vi "Assign LS Slave Timing.vi"(8 "error in (no error)":errorcluster, 10 "MasterTimingInfo":T1, 11 "DAQ Task in":refnum<class "DAQ Task.lvclass">) -> (0 "error out":errorcluster, 3 "DAQ Task out":refnum<class "DAQ Task.lvclass">)   [LabVIEW 2012, in "Data Acquisition.lvlib" / "DAQ Task.lvclass"]
uses:
  DAQ Task.lvclass
  Controls/Master Timing Info.ctl
  DAQ Task.lvclass/DAQ Task.ctl
  <vilib>/DAQmx/configure/trigger.llb/DAQmx Start Trigger (Digital Edge).vi
  <resource>/objmgr/daqmx.rc
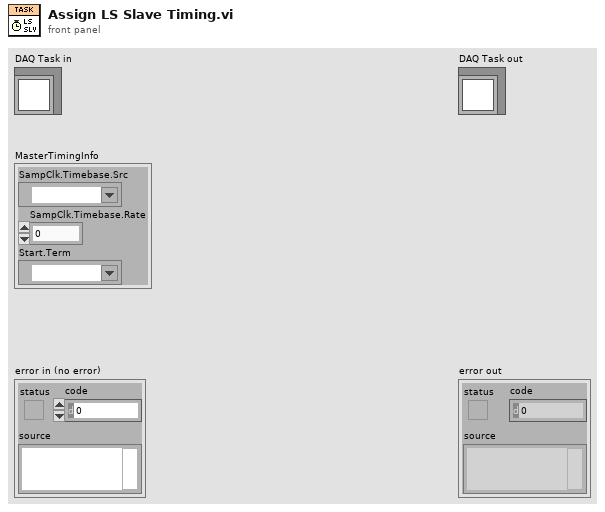
[diagram p1: front panel]
types:
  T1 = typedef "Data Acquisition.lvlib/DAQ Task.lvclass/Master Timing Info.ctl" = cluster{"SampClk.Timebase.Src":tag, "SampClk.Timebase.Rate":dbl, "Start.Term":tag}
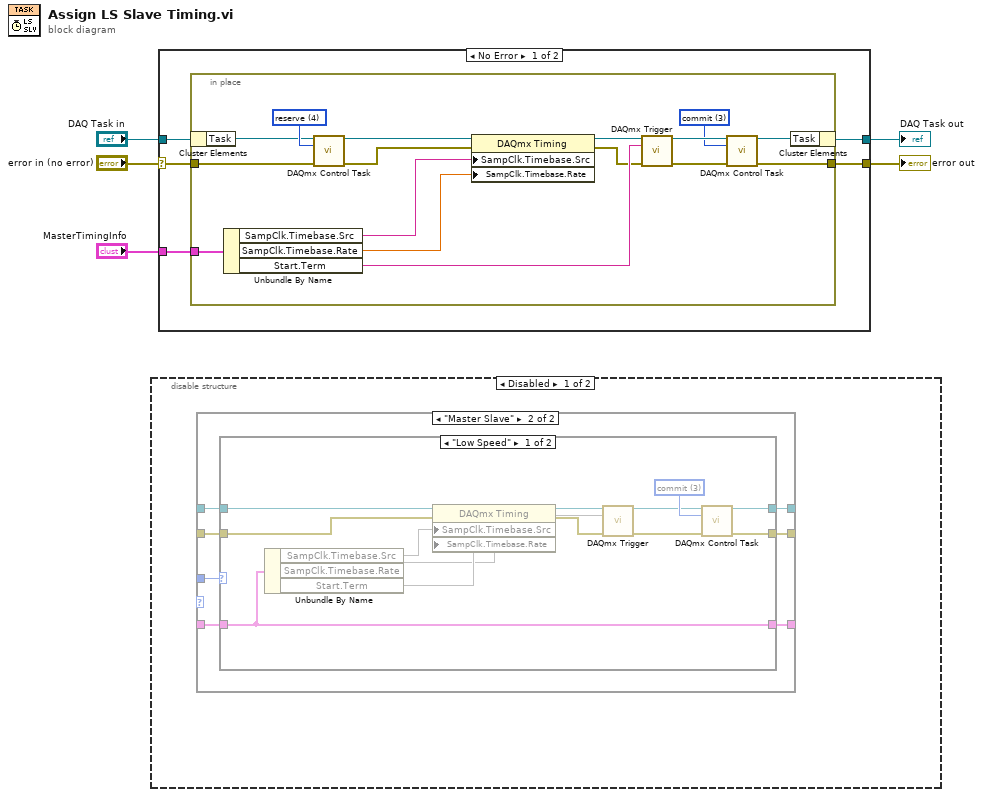
[diagram p0: block diagram]
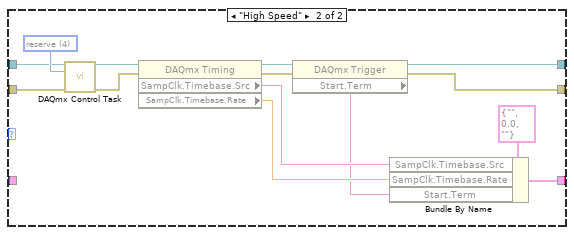
[diagram p3: hidden frame]
diagram:
  n1 = disable-structure shown="Disabled" {
    frame Disabled {
      n2 = case shown="\"Master Slave\"" {
        selector: _ -> [_ _]
        tunnel: [w7 w15] -> _
        tunnel: _ -> [w6 w14]
        tunnel: [w6 w13] -> _
        tunnel: _ -> [w8 w12]
        tunnel: _ -> [w7 w11]
        tunnel: [w8 w10] -> _
        tunnel: _ -> [_ w9]
        frame Default {
        }
        frame "Master Slave" {
          n3 = case shown="\"Low Speed\"" w9 {
            tunnel: w12 -> [w20 w41]
            tunnel: w11 -> [w19 w40]
            tunnel: [w18 w39] -> w10
            tunnel: [w17 w38] -> w15
            tunnel: [w16 w29] -> w13
            tunnel: w14 -> [w16 _]
            frame "Low Speed" {
              w28 = 3 items=["verify"=2, "reserve"=4, "commit"=3, "unreserve"=5, "abort"=6] ("action")
              n4 = Unbundle By Name(w16) -> ("SampClk.Timebase.Src"=w23, "SampClk.Timebase.Rate"=w21, "Start.Term"=w22)
              n5 = property class="DAQmx Timing"(reference=w20, error in=w19, "SampClk.Timebase.Src"=w23, "SampClk.Timebase.Rate"=w21) -> (reference out=w25:refnum<k21>, error out=w24:errorcluster)
              n6 = call-poly <vilib>:"DAQmx Trigger.vi"("task/channels in"=w25, "source"=w22, "error in"=w24) -> ("task out"=w27:refnum<k21>, "error out"=w26:errorcluster)  [unwired: 11 in]
              n7 = call <vilib>:"DAQmx Control Task.vi"("task/channels in"=w27, "action"=w28, "error in"=w26) -> ("task out"=w18:refnum<k21>, "error out"=w17:errorcluster)  [unwired: 11 in]
            }
            frame "High Speed" {
              w42 = 4 items=["verify"=2, "reserve"=4, "commit"=3, "unreserve"=5, "abort"=6] ("action")
              n8 = call <vilib>:"DAQmx Control Task.vi"("task/channels in"=w41, "action"=w42, "error in"=w40) -> ("task out"=w37:refnum<k21>, "error out"=w34:errorcluster)  [unwired: 11 in]
              n9 = property class="DAQmx Timing"(reference=w37, error in=w34) -> (reference out=w36:refnum<k21>, error out=w35:errorcluster, "SampClk.Timebase.Src"=w32:tag, "SampClk.Timebase.Rate"=w31:dbl)
              n10 = property class="DAQmx Trigger"(reference=w36, error in=w35) -> (reference out=w39:refnum<k21>, error out=w38:errorcluster, "Start.Term"=w30:tag)
              n11 = Bundle By Name(cluster=T1 {"SampClk.Timebase.Src"="", "SampClk.Timebase.Rate"=0.0, "Start.Term"=""} ("MasterTimingInfo"), "SampClk.Timebase.Src"=w32, "SampClk.Timebase.Rate"=w31, "Start.Term"=w30) -> (w29:T1)
            }
          }
        }
      }
    }
    frame Enabled {
    }
  }
  n12 = case shown="No Error" "error in (no error)" {
    selector: "error in (no error)" -> [w43 w65]
    tunnel: [w47 w65] -> w5
    tunnel: [w45 w64] -> w4
    tunnel: "DAQ Task in" -> [w44 w64]
    tunnel: "MasterTimingInfo" -> [w46 _]
    frame No Error {
      n13 = in-place {
        in-place-border: [w52] -> w47
        in-place-border: w46 -> [w51]
        in-place-border: w43 -> [w50]
        w55 = 3 items=["verify"=2, "reserve"=4, "commit"=3, "unreserve"=5, "abort"=6] ("action")
        w63 = 4 items=["verify"=2, "reserve"=4, "commit"=3, "unreserve"=5, "abort"=6] ("action")
        n14 = in-place-cluster #1(w44) -> ("Task"=w49:refnum<k21>)
        n15 = Unbundle By Name(w51) -> ("SampClk.Timebase.Src"=w60:tag, "SampClk.Timebase.Rate"=w62:dbl, "Start.Term"=w61:tag)
        n16 = call <vilib>:"DAQmx Control Task.vi"("task/channels in"=w49, "action"=w63, "error in"=w50) -> ("task out"=w54:refnum<k21>, "error out"=w53:errorcluster)  [unwired: 11 in]
        n17 = property class="DAQmx Timing"(reference=w54, error in=w53, "SampClk.Timebase.Src"=w60, "SampClk.Timebase.Rate"=w62) -> (reference out=w58:refnum<k21>, error out=w59:errorcluster)
        n18 = call-poly <vilib>:"DAQmx Trigger.vi"("task/channels in"=w58, "source"=w61, "error in"=w59) -> ("task out"=w56:refnum<k21>, "error out"=w57:errorcluster)  [unwired: 11 in]
        n19 = call <vilib>:"DAQmx Control Task.vi"("task/channels in"=w56, "action"=w55, "error in"=w57) -> ("task out"=w48:refnum<k21>, "error out"=w52:errorcluster)  [unwired: 11 in]
        n20 = in-place-cluster #1("Task"=w48) -> (w45:refnum<class "DAQ Task.lvclass">)
      }
    }
    frame Error {
    }
  }
  "error out" <- w5
  "DAQ Task out" <- w4
